vi "Perform Audio Measurements.vi"(0 "Measurement Configuration":T1={"Band start"=20.0, "Band stop"=20000.0, "Weighting filter"="", "Amplitude"=1.0, "Frequency"=1000.0, "Full scale range"=3.16, "Analog source resource name"="", "Protocol capture resource name"="", "Data line"=0, "Sample rate"=12288000.0, "Measurement duration"=19200.0, "Channel"="0L", "Frame sync edge for channel 0"=0, "Channel count per frame"=2, "Channel length"=32, "Bit depth"=24, "Channel 0 offset"=1, "Endianness"=0, "Data justification"=0, "Frame length"=64, "Frame sync pulse width"=32, "Bit clock edge sync"=1} {"Sample rate" format="%#.0f"}, 1 "I2S waveforms":waveform(dbl)[](array[waveform]), 3 "error in":errorcluster) -> (7 "Measurement Results":T2, 10 "error out":errorcluster)   [LabVIEW 2021, in "audio_adc_acDualChannelMeasurement.lvlib"]
uses:
  audio_adc_acDualChannelMeasurement.lvlib
  Measurement Results.ctl
  Measurement Configuration.ctl
  <vilib>/addons/_NISVFA/_Shared subVIs/Controls/svc_Window.ctl
  <vilib>/addons/_NISVFA/_Shared subVIs/Common/SVL Set dB Reference (N Ch - 1 Ref).vi
  <vilib>/addons/Sound and Vibration/svt_Level/SVL AC & DC Level (Time) (N Ch).vi
  <vilib>/addons/Sound and Vibration/svt_Single Tone Measurements/SVT Spurious Free Dynamic Range (Frequency) (1 Ch).vi
  <vilib>/addons/_NISVFA/_Spectrum Processing/SVFA Unit Conversion (Complex) (1 Ch).vi
  <vilib>/addons/_NISVFA/_Shared subVIs/Common/SVL Set dB Reference (1 Ch).vi
  <vilib>/addons/Sound and Vibration/svt_Level/SVL AC & DC Level (Time) (1 Ch).vi
  <vilib>/addons/_NISVFA/_Spectrum Processing/SVFA Get Spectrum Subset.vi
  <vilib>/addons/_NISVFA/_Spectrum Processing/SVFA Get Spectrum Subset (Complex) (1 Ch).vi
  <vilib>/addons/_NISVFA/_Shared subVIs/Common/svc_Window Parameters.vi
  <vilib>/addons/_NISVFA/_Shared subVIs/Common/svc_Extract Single Tone Information (complex).vi
  <vilib>/addons/_NISVFA/_Shared subVIs/Common/svc_Check Frequency Range in Spectrum.vi
  <vilib>/addons/_NISVFA/_Spectrum Processing/SVFA Spectrum Peak Search.vi
  <vilib>/addons/_NISVFA/_Spectrum Processing/SVFA Spectrum Peak Search (1 Ch).vi
  <vilib>/addons/_NISVFA/_Shared subVIs/Common/svc_Spectrum Units.vi
  <vilib>/addons/_NISVFA/_Shared subVIs/Common/svc_Log View for Spectrum (1Ch).vi
  <vilib>/addons/_NISVFA/_Spectrum Processing/SVFA Unit Conversion (1 Ch).vi
  <vilib>/addons/_NISVFA/_Shared subVIs/Common/svc_Complex Datatype Defaults.vi
  <vilib>/addons/_NISVFA/_Shared subVIs/Common/svc_Build Unit Label for Frequency Range.vi
  <vilib>/addons/_NISVFA/_Shared subVIs/Common/SVL Set dB Reference (variant).vi
  <vilib>/addons/_NISVFA/_Shared subVIs/Common/svc_Get SV Channel Info.vi
  <vilib>/Analysis/baseanly.llb/Mean.vi
  <vilib>/Analysis/baseanly.llb/Mean (DBL).vi
  <vilib>/addons/_NISVFA/_Shared subVIs/Windowing/svfa_Scaled Time Domain Window (Array).vi
  <vilib>/addons/_NISVFA/_Spectrum Processing/SVFA Get Tone Amplitude and Phase (1 Ch).vi
  <vilib>/addons/_NISVFA/_Spectrum Processing/subVIs/svfa_Compute Complex Spectrum for Export.vi
  <vilib>/addons/_NISVFA/_Shared subVIs/Common/svc_Check Frequency Range in Bandwidth.vi
  <vilib>/addons/_NISVFA/_Shared subVIs/Common/svc_Convert Start and Stop to Start Index and Length.vi
  <vilib>/addons/_NISVFA/_Spectrum Processing/subVIs/svfa_Spectrum Peak Search.vi
  <vilib>/addons/_NISVFA/_Shared subVIs/Common/svc_Format Value (DBL).vi
  <vilib>/addons/_NISVFA/_Shared subVIs/Common/svc_Get Weighting Enum and Labels.vi
  <vilib>/addons/_NISVFA/_Shared subVIs/Common/svc_Engineering Units to Unit Label.vi
  <vilib>/addons/_NISVFA/_Shared subVIs/Common/svc_Surround NonAlpha String with Parentheses.vi
  <vilib>/dlg_ctls.llb/Space Constant.vi
  <vilib>/addons/_NISVFA/_Shared subVIs/Common/svc_Unwrap Phase.vi
  <vilib>/addons/_NISVFA/_Shared subVIs/Common/svc_Convert Spectrum Array to dB.vi
  <vilib>/addons/_NISVFA/_Spectrum Processing/subVIs/svfa_Conversion Utility (spectrum info).vi
  <vilib>/addons/_NISVFA/_Shared subVIs/Common/svc_Unit Label to Engineering Units.vi
  <vilib>/addons/_NISVFA/_Spectrum Processing/subVIs/svfa_Spectrum Info Window to windowTd Type Def.vi
  <vilib>/Analysis/4window.llb/Force Window.vi
  <vilib>/Analysis/4window.llb/Force Window (DBL).vi
  <vilib>/Analysis/4window.llb/Exponential Window.vi
  <vilib>/Analysis/4window.llb/Exponential Window (DBL).vi
  <vilib>/addons/_NISVFA/_Spectrum Processing/subVIs/svfa_Window Frequency Response.vi
  <vilib>/addons/_NISVFA/_Spectrum Processing/subVIs/svfa_Window Frequency Response (double array).vi
  <vilib>/Analysis/baseanly.llb/Dot Product.vi
  <vilib>/Analysis/baseanly.llb/Complex Dot Product.vi
  <vilib>/addons/_NISVFA/_Spectrum Processing/subVIs/svfa_Peak Rough Search Indices.vi
  <vilib>/addons/_NISVFA/_Shared subVIs/Common/svc_Unit Label Lexical Class.vi
  <vilib>/addons/_NISVFA/_Spectrum Processing/subVIs/svfa_Peak to RMS to Peak2Peak.vi
  <vilib>/addons/_NISVFA/_Spectrum Processing/subVIs/svfa_Mag to Mag2.vi
  <vilib>/addons/_NISVFA/_Spectrum Processing/subVIs/svfa_Linear to dB.vi
  <vilib>/addons/_NISVFA/_Spectrum Processing/subVIs/svfa_dBrefA to dBrefB.vi
  <vilib>/addons/_NISVFA/_Spectrum Processing/subVIs/svfa_Spectrum to Spectral Density.vi
  <vilib>/addons/_NISVFA/_Spectrum Processing/subVIs/svfa_Rect Window Frequency Response.vi
  <vilib>/addons/_NISVFA/_Spectrum Processing/subVIs/svfa_Cosine Window Coefficients.vi
  <vilib>/addons/Sound and Vibration/svt_Weighting/SVT Weighting Filter (N Ch).vi
  <vilib>/addons/_NISVFA/_Shared subVIs/Common/svc_Caller VI Returned in Error Source.vi
  <vilib>/addons/_NISVFA/_Shared subVIs/Common/svc_Get Window Info.vi
  <vilib>/Analysis/0measdsp.llb/Scaled Time Domain Window.vi
  <vilib>/Analysis/0measdsp.llb/Scaled Time Domain Window (DBL).vi
  <vilib>/Utility/error.llb/Error Cluster From Error Code.vi
  <vilib>/Analysis/baseanly.llb/Std Deviation and Variance.vi
  <vilib>/addons/Sound and Vibration/svt_Single Tone Measurements/SVT Gain (Time) (1 Ch).vi
  <vilib>/addons/Sound and Vibration/svt_Distortion/SVT SNR without Harmonics (Frequency) (1 Ch).vi
  <vilib>/addons/Sound and Vibration/svt_Single Tone Measurements/SVT Dynamic Range (Frequency) (1 Ch).vi
  <vilib>/addons/Sound and Vibration/svt_Distortion/subVIs/sv_Check Data Valid (Audio) (1 Ch).vi
  <vilib>/addons/_NISVFA/_Shared subVIs/Common/svc_Convert Frequency to Frequency String.vi
  <vilib>/Analysis/4window.llb/window parameters.vi
  <vilib>/Analysis/4window.llb/Window Properties.vi
  <vilib>/Analysis/4window.llb/Window Properties by Name.vi
  <vilib>/addons/_NISVFA/_Spectrum Processing/subVIs/svfa_Spectrum Peak Tone Search and Estimation (complex).vi
  <vilib>/measure/masignal.llb/Tones and Noise Waveform.vi
  <vilib>/addons/_NISVFA/_Shared subVIs/Common/svc_FFT with Window.vi
  <vilib>/Analysis/1siggen.llb/Square Wave.vi
  <vilib>/addons/_NISVFA/_Spectrum Processing/subVIs/svfa_Three Finger Peak Search.vi
  <vilib>/addons/Sound and Vibration/svt_Distortion/subVIs/sv_Peak View Amplitude (1 Ch).vi
  <vilib>/addons/Sound and Vibration/svt_Single Tone Measurements/SoundVib_SingleTone.lvlib
  <vilib>/addons/Sound and Vibration/svt_Distortion/SoundVib_Distortion.lvlib
  <vilib>/addons/Sound and Vibration/svt_Weighting/SoundVib_ABCWeighting.lvlib
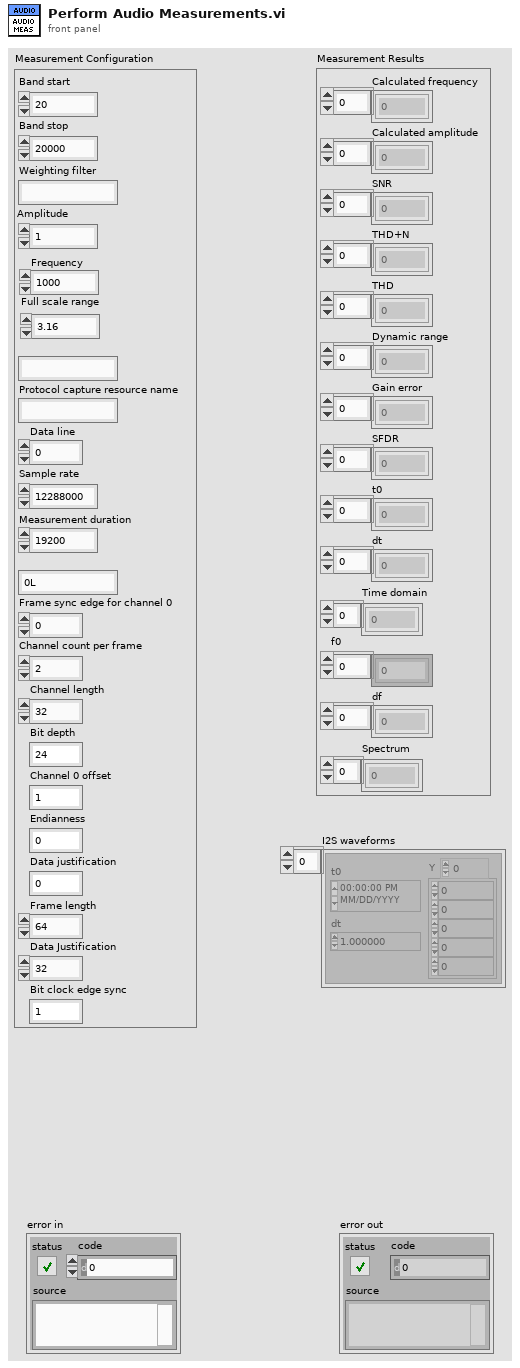
[diagram p1: front panel]
types:
  T1 = typedef "audio_adc_acDualChannelMeasurement.lvlib/Measurement Configuration.ctl" = cluster{"Band start":dbl, "Band stop":dbl, "Weighting filter":string, "Amplitude":dbl, "Frequency":dbl, "Full scale range":dbl, "Analog source resource name":string, "Protocol capture resource name":string, "Data line":u16, "Sample rate":dbl, "Measurement duration":dbl, "Channel":string, "Frame sync edge for channel 0":u32, "Channel count per frame":u32, "Channel length":u32, "Bit depth":u32, "Channel 0 offset":u32, "Endianness":u32, "Data justification":u32, "Frame length":u32, "Frame sync pulse width":u32, "Bit clock edge sync":u32}
  T2 = typedef "audio_adc_acDualChannelMeasurement.lvlib/Measurement Results.ctl" = cluster{"Calculated frequency":dbl[], "Calculated amplitude":dbl[], "SNR":dbl[], "THD+N":dbl[], "THD":dbl[], "Dynamic range":dbl[], "Gain error":dbl[], "SFDR":dbl[], "t0":dbl[], "dt":dbl[], "Time domain":dbl[], "f0":dbl[], "df":dbl[], "Spectrum":dbl[]}
  T3 = cluster{"start frequency":dbl, "stop frequency":dbl}
  T4 = typedef "svc_Window.ctl" = u32
  T5 = enum16{"no change", "spectrum", "spectral density"}
  T6 = cluster{"linear/dB":enum16{"no change", "linear", "dB"}, "dB reference (0: no change)":dbl, "power/magnitude":enum16{"no change", "power", "magnitude"}, "view":enum16{"no change", "rms", "peak", "peak-peak"}}
  T7 = cluster{"gain units":enum16{"dB", "linear ratio"}, "detected fundamental amplitude units":enum16{"EU rms", "EU peak", "EU peak-peak"}}
  T8 = cluster{"SNR units":enum16{"dB", "linear ratio", "%"}, "detected fundamental amplitude units":enum16{"EU rms", "EU peak", "EU peak-peak"}}
  T9 = typedef "svc_Spectrum Info.ctl" = cluster{"channel name":string, "description":string, "x-axis units":T10, "spectral info":cluster{"spectrum type":T11, "linear/dB":enum16{"linear", "dB"}, "window":u16, "window size":i32, "FFT size":i32}, "engineering units":T12, "custom label":string, "dB reference [EU]":dbl, "peak units":enum16{"rms", "peak", "peak-peak"}, "weighting filter":T13, "spectral density?":bool, "unit label":string, "spectrum skewed?":bool, "complimentary spectrum units":T14}
  T10 = typedef "svc_X-Axis Units.ctl" = u16
  T11 = typedef "svc_Spectrum Type.ctl" = enum16{"FFT Spectrum [complex]", "Amplitude [Magnitude]", "Power [Magnitude^2]", "Cross Spectrum [complex]", "Frequency Response [Complex]"}
  T12 = typedef "svc_Engineering Units Text Ring.ctl" = u16
  T13 = typedef "svc_Weighting Filter Text Ring.ctl" = u16
  T14 = typedef "svc_Complimentary Spectrum Units.ctl" = enum16{"none", "radians", "degrees", "cycles", "imaginary"}
  T15 = cluster{"complex spectrum response":cluster{"f0":dbl, "df":dbl, "complex spectrum":cdb[]}, "spectrum info":T9}
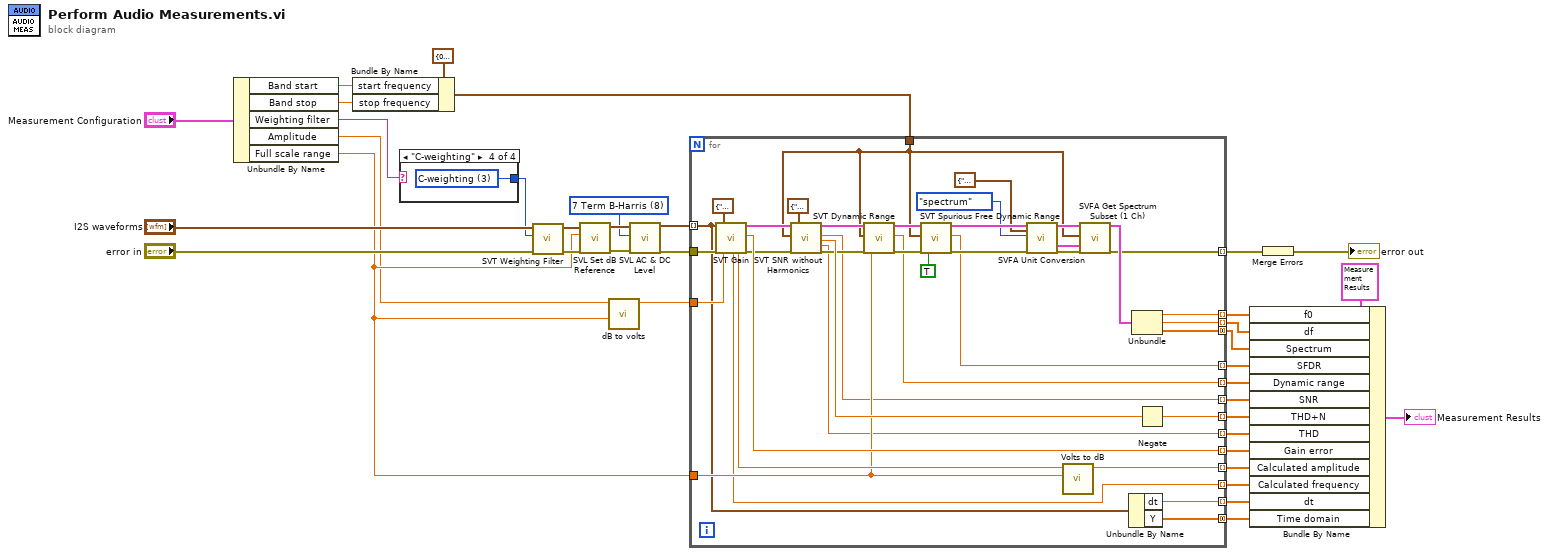
[diagram p0: block diagram]
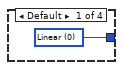
[diagram p2: hidden frame]
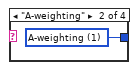
[diagram p3: hidden frame]
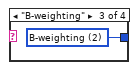
[diagram p4: hidden frame]
diagram:
  w22 = T4 8 items=["None"=0, "Hanning"=1, "Hamming"=2, "Blackman-Harris"=3, "Exact Blackman"=4, "Blackman"=5, "Flat Top"=6, "4 Term B-Harris "=7, "7 Term B-Harris"=8, "Low Sidelobe"=9, "Force"=64, "Exponential"=65, "Blackman Nuttall"=11, "Triangle"=30, "Bartlett-Hanning"=31, "Bohman"=32, "Parzen"=33, "Welch"=34, "Kaiser"=60, "Dolph-Chebyshev"=61, "Gaussian"=62] ("window")
  n1 = Unbundle By Name("Measurement Configuration") -> ("Band start"=w30:dbl, "Band stop"=w31:dbl, "Weighting filter"=w13:string, "Amplitude"=w11:dbl, "Full scale range"=w12:dbl)
  n2 = Bundle By Name(cluster=T3 {"start frequency"=0.0, "stop frequency"=0.0} ("frequency range"), "start frequency"=w30, "stop frequency"=w31) -> (w16:T3)
  n3 = case shown="\"C-weighting\"" w13 {
    tunnel: [w37 w38 w39 w40] -> w10
    frame Default {
      w37 = u16 0 items=["Linear", "A-weighting", "B-weighting", "C-weighting"] ("weighting")
    }
    frame "A-weighting" {
      w38 = u16 1 items=["Linear", "A-weighting", "B-weighting", "C-weighting"] ("weighting")
    }
    frame "B-weighting" {
      w39 = u16 2 items=["Linear", "A-weighting", "B-weighting", "C-weighting"] ("weighting")
    }
    frame "C-weighting" {
      w40 = u16 3 items=["Linear", "A-weighting", "B-weighting", "C-weighting"] ("weighting")
    }
  }
  n4 = call-poly <vilib>:"SVT Weighting Filter.vi"("error in (no error)"="error in", "weighting"=w10, "scaled signals [EU]"="I2S waveforms") -> ("error out"=w27:errorcluster, "weighted signals [EU]"=w26:waveform(dbl)[])  [unwired: 6 in]
  n5 = call-poly <vilib>:"SVL Set dB Reference.vi"("error in (no error)"=w27, "dB reference [EU]"=w12, "scaled signals in [EU]"=w26) -> ("error out"=w23:errorcluster, "scaled signals out [EU]"=w24:waveform(dbl)[])  [unwired: 7 in]
  n6 = call "dB to volts.vi"("Full scale range"=w12, "Voltage(dB)"=w11) -> ("Voltage(volts)"=w17:dbl)  [unwired: 9 in]
  n7 = call-poly <vilib>:"SVL AC & DC Level.vi"("scaled signals in [EU]"=w24, "window"=w22, "error in (no error)"=w23) -> ("AC signals [EU]"=w2:waveform(dbl)[], "error out"=w25:errorcluster)  [unwired: 11 in, 4 out]
  n8 = for {
    tunnel: [w78] -> w35 mode=concatenating
    tunnel: [w77] -> w34 mode=indexing
    tunnel: [w76] -> w33 mode=indexing
    tunnel: [w60] -> w20 mode=indexing
    tunnel: [w59] -> w19 mode=indexing
    tunnel: [w58] -> w18 mode=concatenating
    tunnel: w17 -> [w57]
    tunnel: w16 -> [w54]
    tunnel: w12 -> [w49]
    tunnel: [w48] -> w9 mode=indexing
    tunnel: [w47] -> w8 mode=indexing
    tunnel: [w46] -> w7 mode=indexing
    tunnel: [w45] -> w6 mode=indexing
    tunnel: [w44] -> w5 mode=indexing
    tunnel: [w43] -> w4 mode=indexing
    tunnel: [w42] -> w3 mode=indexing
    tunnel: w2 -> [w41] mode=indexing
    tunnel: w25 -> [w72]
    tunnel: [w52] -> w15 mode=indexing
    n9 = call-poly <vilib>:"SVT Gain.vi"("scaled signal [EU]"=w41, "error in (no error)"=w72, "desired units"=T7 {"gain units"=enum."dB", "detected fundamental amplitude units"=enum."EU peak"}, "amplitude [EU peak]"=w57) -> ("detected fundamental\nfrequency [Hz]"=w42:dbl, "detected fundamental\namplitude"=w56:dbl, "complex spectrum"=w65:T15, "gain"=w76:dbl, "error out"=w66:errorcluster)  [unwired: 10 in, 1 out]
    n10 = call-poly <vilib>:"SVT SNR without Harmonics.vi"("complex spectrum"=w65, "frequency range"=w54, "error in (no error)"=w66, "desired units"=T8 {"SNR units"=enum."dB", "detected fundamental amplitude units"=enum."EU rms"}) -> ("complex spectrum"=w68:T15, "SNR (without harmonics)"=w46:dbl, "SINAD"=w69:dbl, "THD"=w44:dbl, "error out"=w67:errorcluster)  [unwired: 8 in, 3 out]
    n11 = call-poly <vilib>:"SVT Dynamic Range.vi"("complex spectrum"=w68, "frequency range"=w54, "error in (no error)"=w67, "full scale amplitude [EU peak]"=w49) -> ("dup complex spectrum"=w73:T15, "dynamic range"=w47:dbl, "error out"=w74:errorcluster)  [unwired: 10 in, 3 out]
    n12 = call-poly <vilib>:"SVT Spurious Free Dynamic Range.vi"("complex spectrum"=w73, "frequency range"=w54, "error in (no error)"=w74, "exclude harmonics"=TRUE) -> ("complex spectrum"=w63:T15, "spurious free dynamic range"=w48:dbl, "error out"=w64:errorcluster)  [unwired: 8 in, 5 out]
    n13 = call-poly <vilib>:"SVFA Unit Conversion.vi"("complex spectrum"=w63, "desired scaling"=T6 {"linear/dB"=enum."dB", "dB reference (0: no change)"=0.0, "power/magnitude"=enum."magnitude", "view"=enum."peak-peak"}, "spectral density desired"=T5."spectrum", "error in (no error)"=w64) -> ("converted spectrum"=w55:cluster{"x0":dbl, "dx":dbl, "magnitude":dbl[]}, "spectrum info out"=w51:T9, "error out"=w50:errorcluster)  [unwired: 10 in, 3 out]
    n14 = call "Volts to dB.vi"("Full scale range"=w49, "Voltage(V)"=w56) -> ("Voltage(dB)"=w43:dbl)  [unwired: 9 in]
    n15 = call <vilib>:"SVFA Get Spectrum Subset (1 Ch).vi"("spectrum"=w55, "range"=w54, "spectrum info"=w51, "error in (no error)"=w50) -> ("spectrum subset"=w53:cluster{"x0":dbl, "dx":dbl, "magnitude":dbl[]}, "error out"=w52:errorcluster)  [unwired: 10 in, 4 out]
    n16 = Unbundle By Name ("Get Waveform Components")(w41) -> ("dt"=w77:dbl, "Y"=w78:dbl[])
    n17 = Unbundle(w53) -> ("x0"=w60:dbl, "dx"=w59:dbl, "magnitude"=w58:dbl[])
    n18 = Negate(x=w69) -> (-x=w45:dbl)
  }
  n19 = Bundle By Name(cluster=T2 {"Calculated frequency"=[], "Calculated amplitude"=[], "SNR"=[], "THD+N"=[], "THD"=[], "Dynamic range"=[], "Gain error"=[], "SFDR"=[], "t0"=[], "dt"=[], "Time domain"=[], "f0"=[], "df"=[], "Spectrum"=[]} ("Measurement Results"), "f0"=w20, "df"=w19, "Spectrum"=w18, "SFDR"=w9, "Dynamic range"=w8, "SNR"=w7, "THD+N"=w6, "THD"=w5, "Gain error"=w33, "Calculated amplitude"=w4, "Calculated frequency"=w3, "dt"=w34, "Time domain"=w35) -> (→"Measurement Results":T2)
  n20 = Merge Errors(w15) -> (→"error out":errorcluster)
